vi "MGCC_main_v2.vi"() -> ()   [LabVIEW 2016]
uses:
  <vilib>/imath/engines/lvmath2/RunTimeEngine/IndexRead/NIMS V(S).vi
  <instcachedir>/0/NIMS V(S)_0488751826AF41519A22953C041130DC.lvgen/NIMS V(S)_0488751826AF41519A22953C041130DC_003.vi
  <vilib>/imathl/engines/lvmath/Functions/Error Handling/Create Error.vi
  <vilib>/imath/engines/lvmath2/RunTimeEngine/NodeEndStatement/NIMS_NodeEndStatement_Output.vi
  <instcachedir>/0/NIMS_NodeEndStatement_Output_53EC0D466D134D7ABD903AC30B43404B.lvgen/NIMS_NodeEndStatement_Output_53EC0D466D134D7ABD903AC30B43404B_011.vi
  <vilib>/imath/engines/lvmath2/RunTimeEngine/ErrorHandling/NIMS_Finalize Error.vi
panel:
  in  "Manual turn off":bool
  in  "Event Manual panel":bool
  out "Function":bool[](array[boolean])
  out "Name_Function":string[](array[string])
  out "State":bool[](array[boolean])
  out "Name of state":string[](array[string])
  out "Current State":string
  out "Next State":string
  out "date/time string":string
  out "Boolean 4":bool
  out "Boolean 3":bool
  out "Boolean 2":bool
  out "Boolean":bool
  in  "Combo Box":string(combo)="State1"
  # "Interrupts"
  # "Finte State Machine"
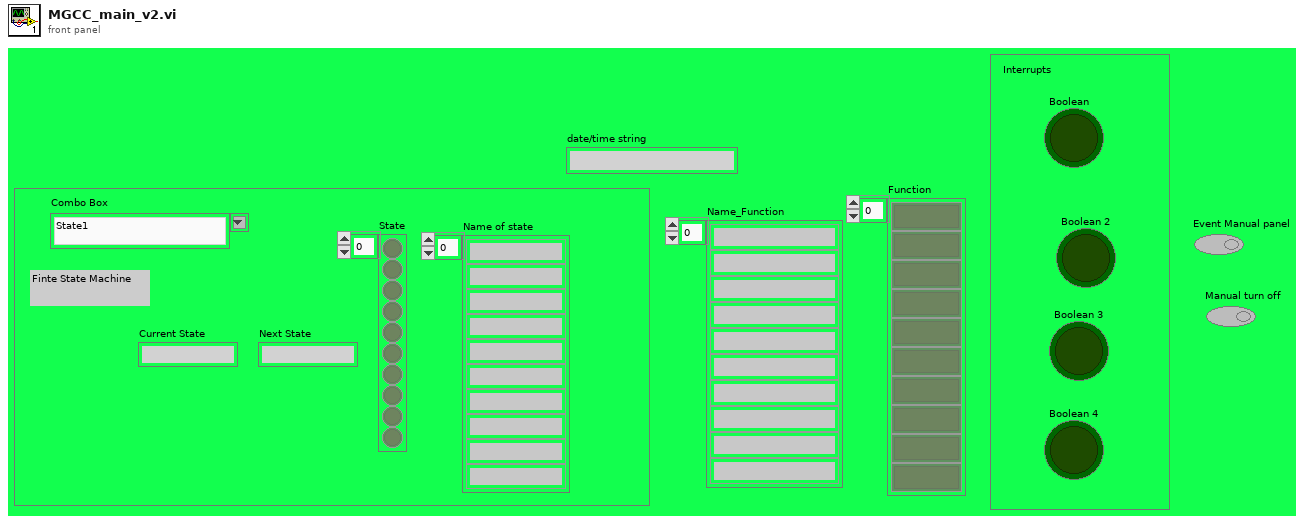
[diagram p1: front panel]
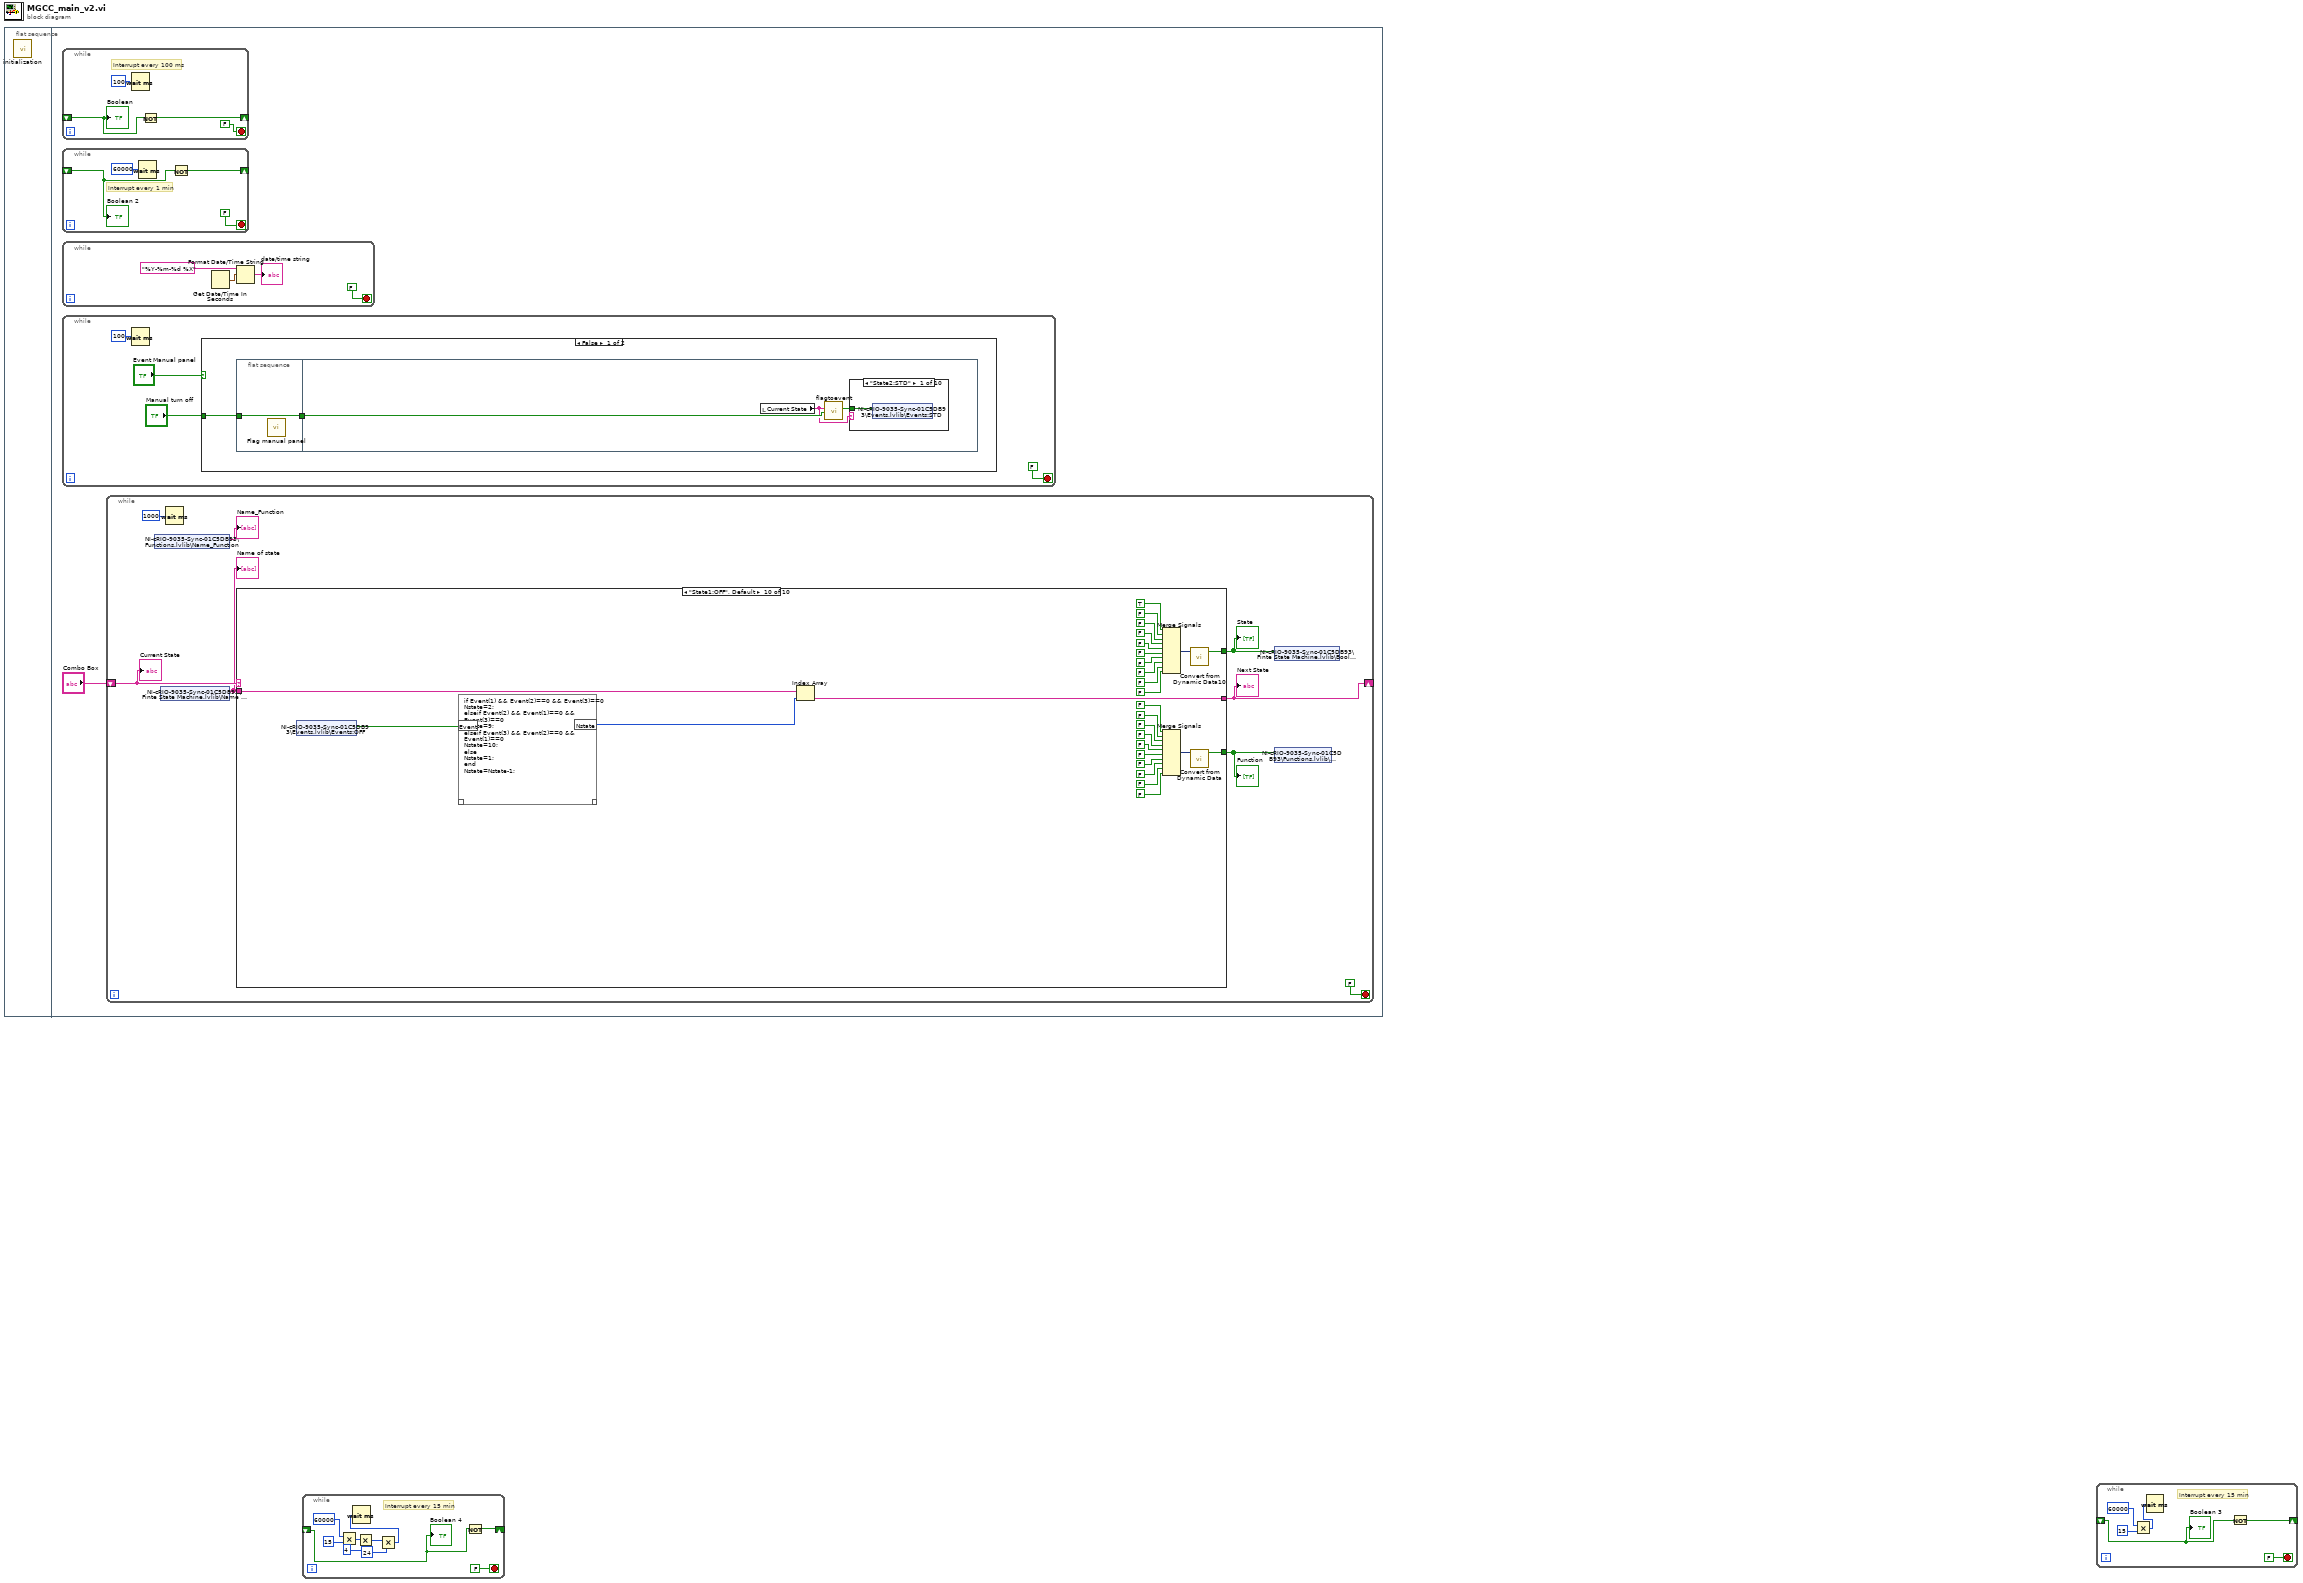
[diagram p0: block diagram]
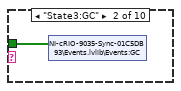
[diagram p2: hidden frame]
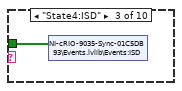
[diagram p3: hidden frame]
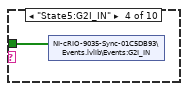
[diagram p4: hidden frame]
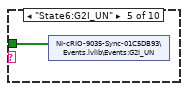
[diagram p5: hidden frame]
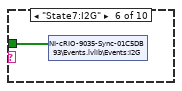
[diagram p6: hidden frame]
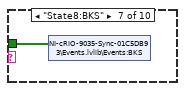
[diagram p7: hidden frame]
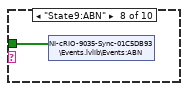
[diagram p8: hidden frame]
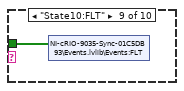
[diagram p9: hidden frame]
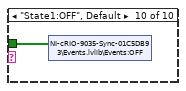
[diagram p10: hidden frame]
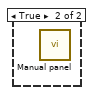
[diagram p11: hidden frame]
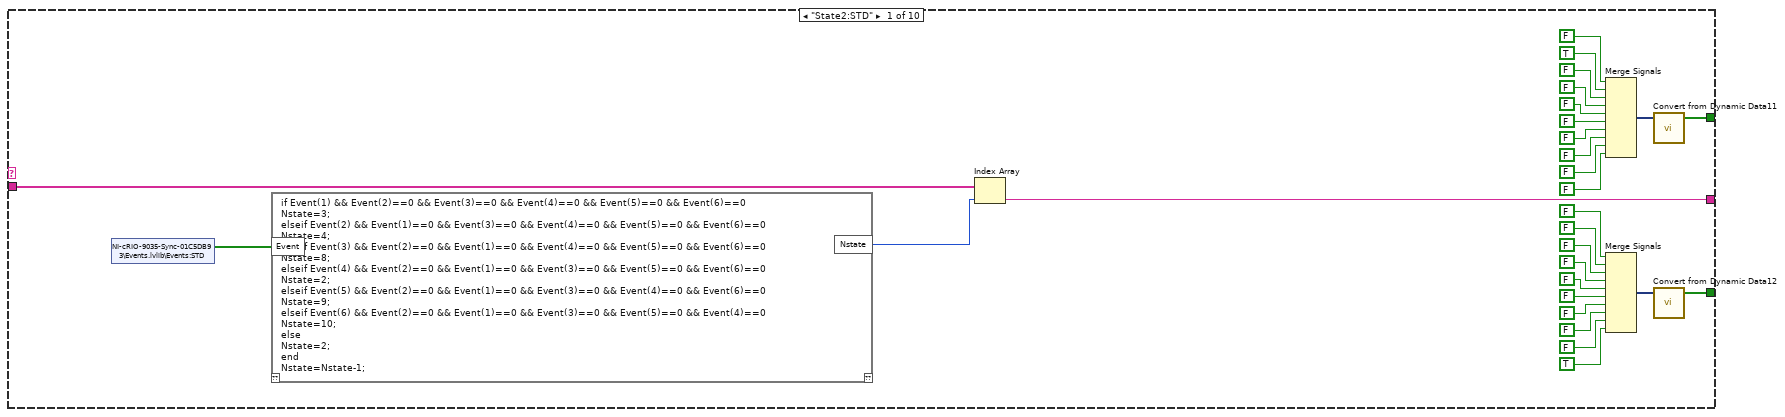
[diagram p12: hidden frame]
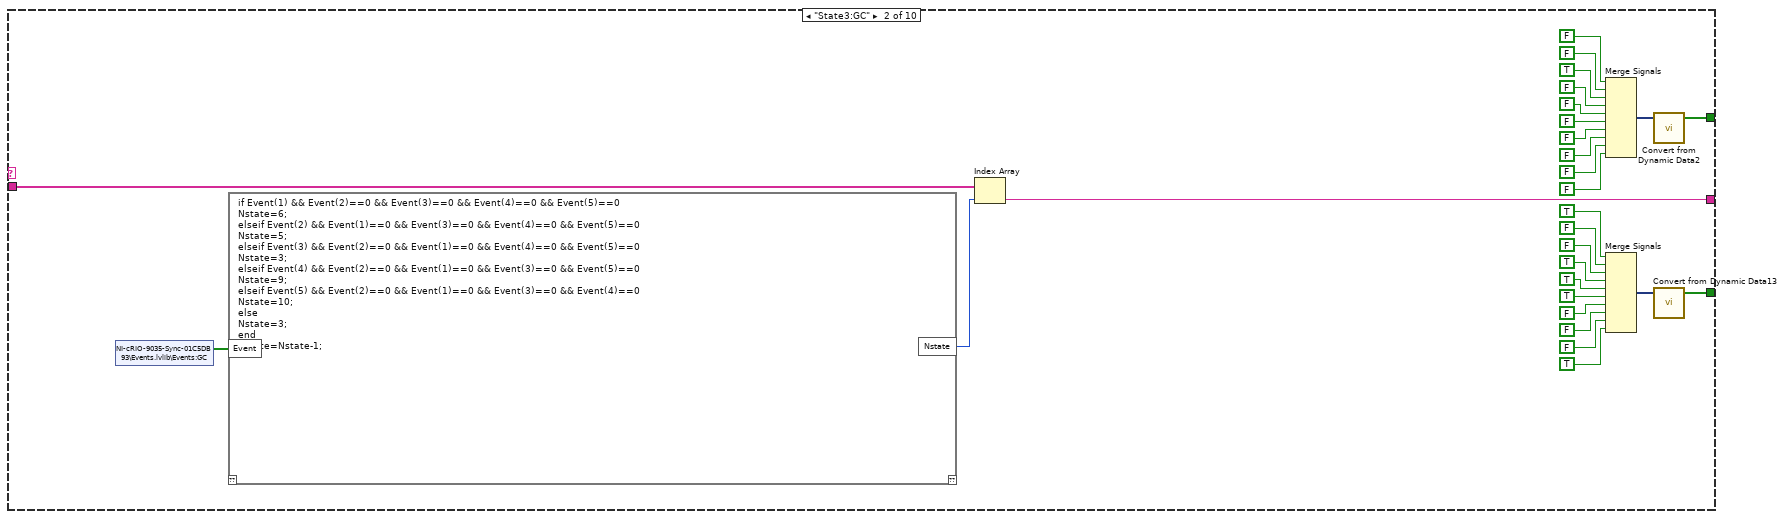
[diagram p13: hidden frame]
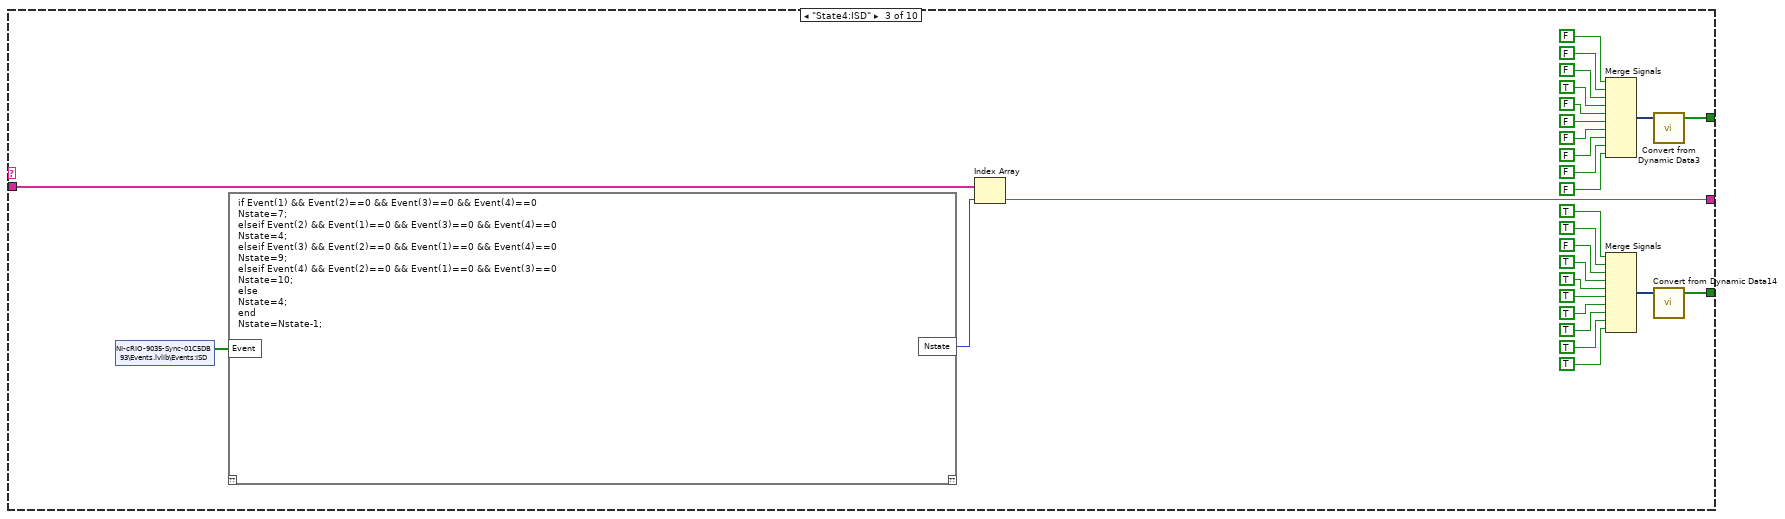
[diagram p14: hidden frame]
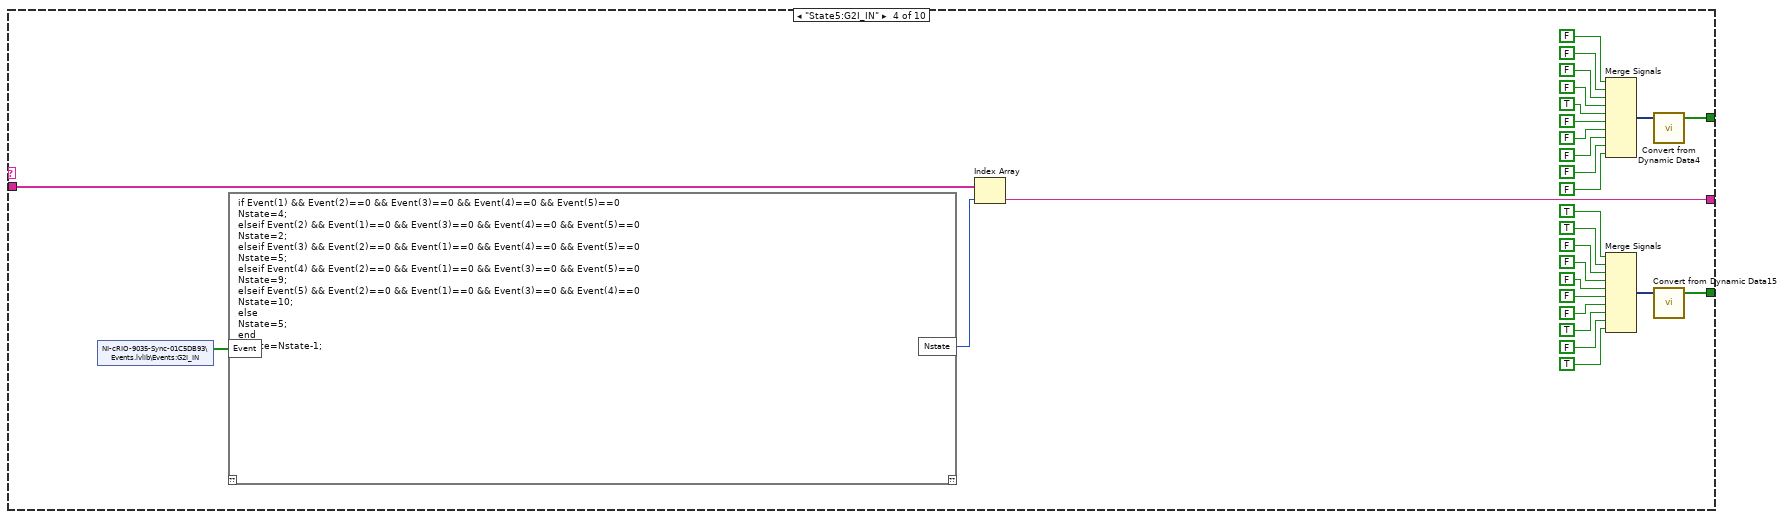
[diagram p15: hidden frame]
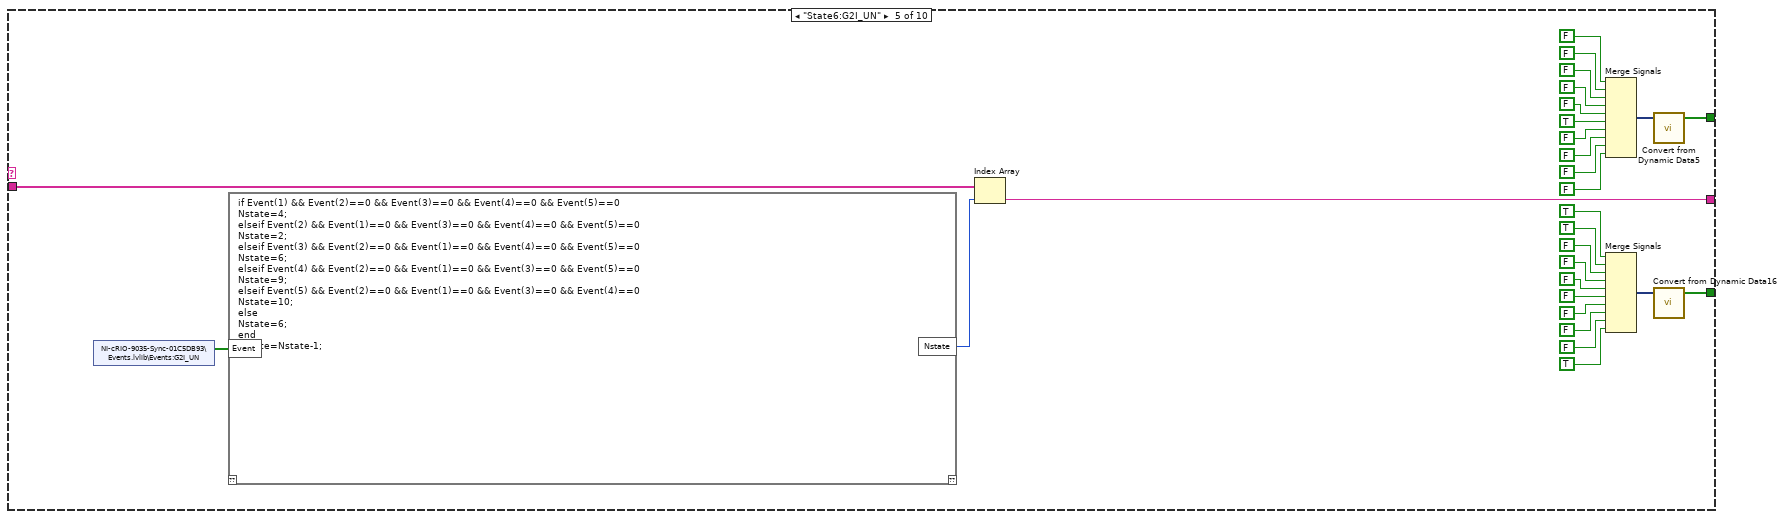
[diagram p16: hidden frame]
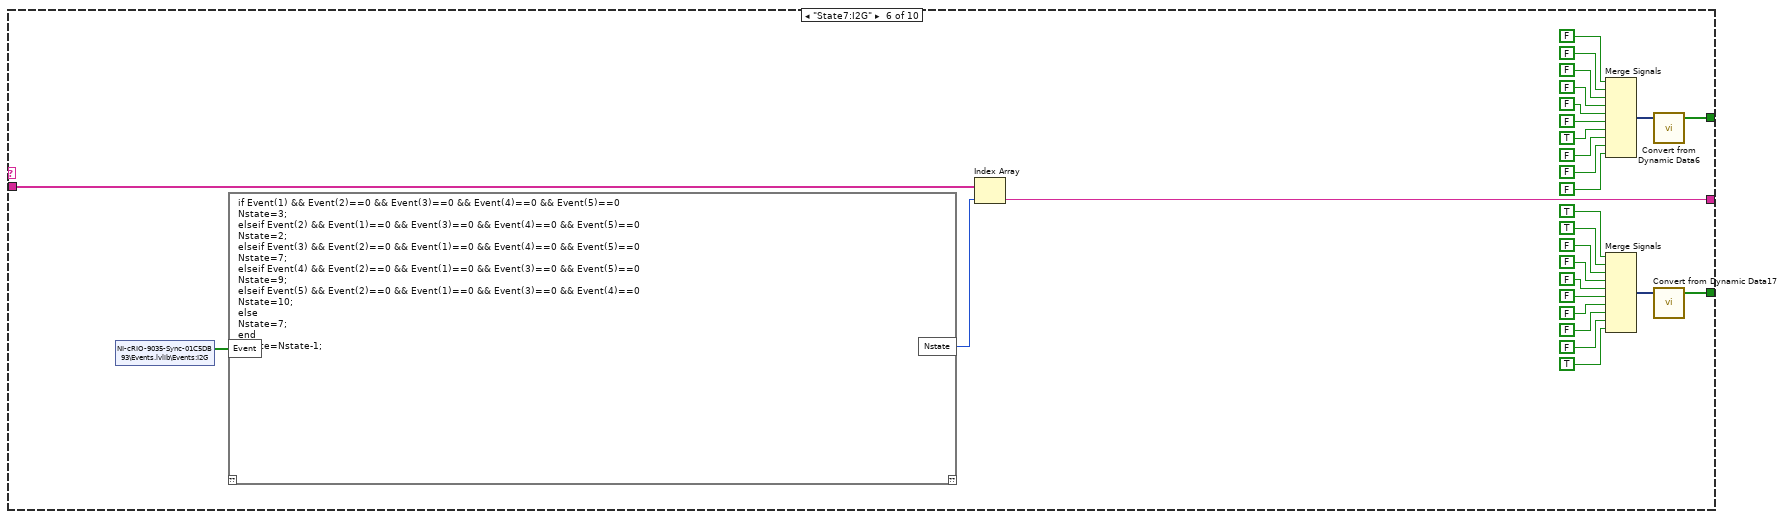
[diagram p17: hidden frame]
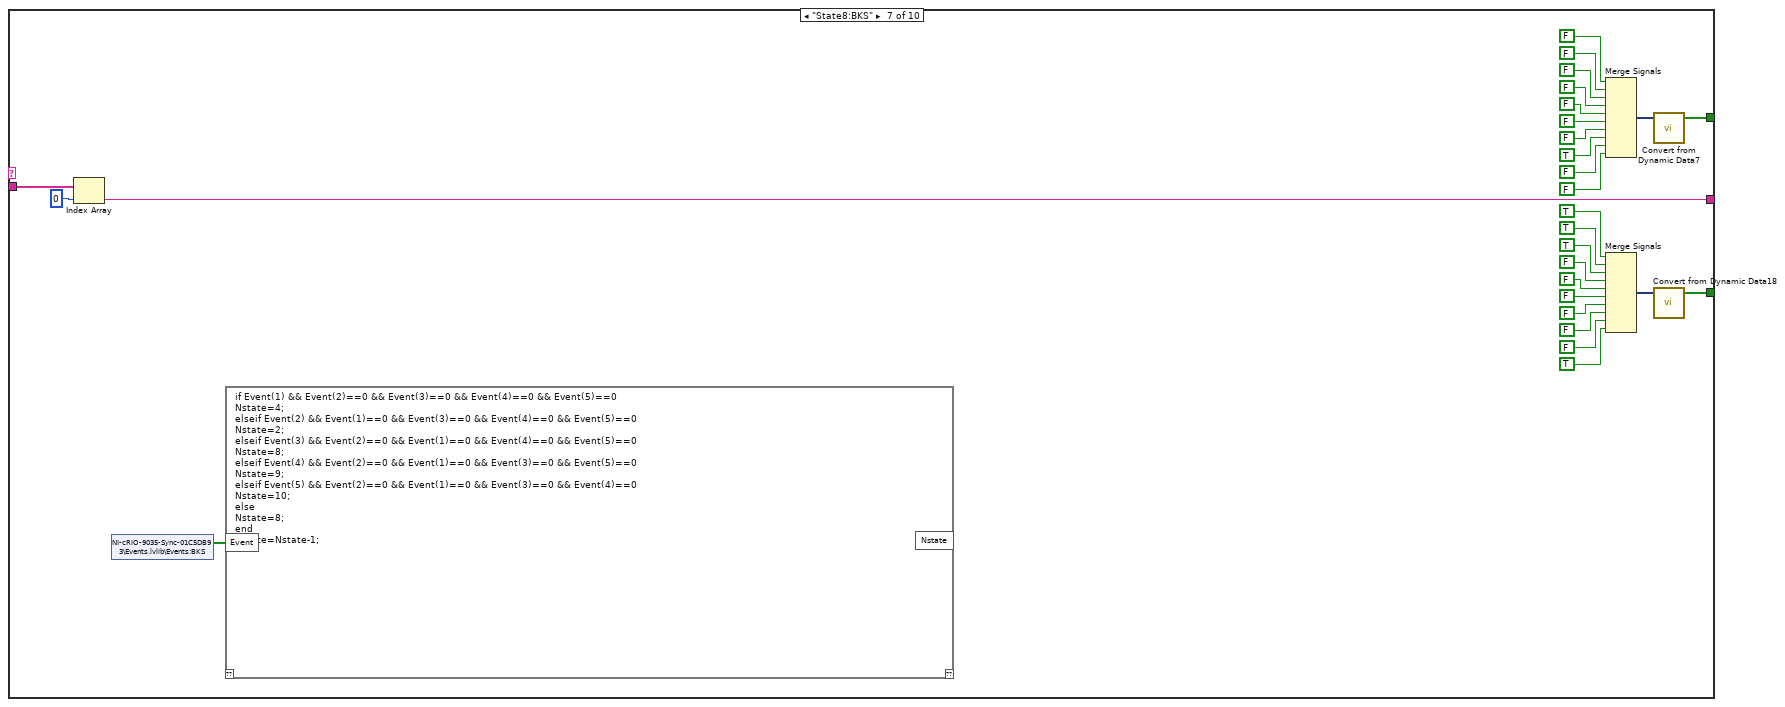
[diagram p18: hidden frame]
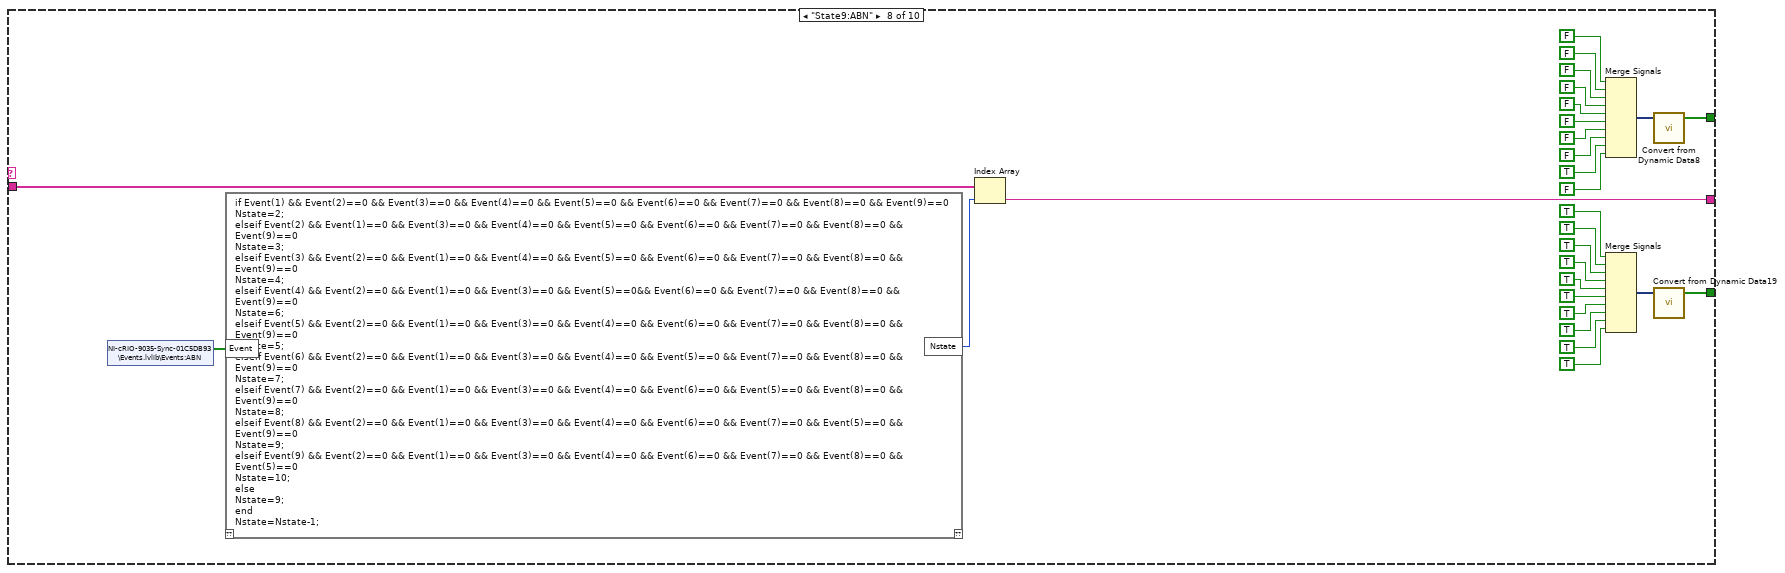
[diagram p19: hidden frame]
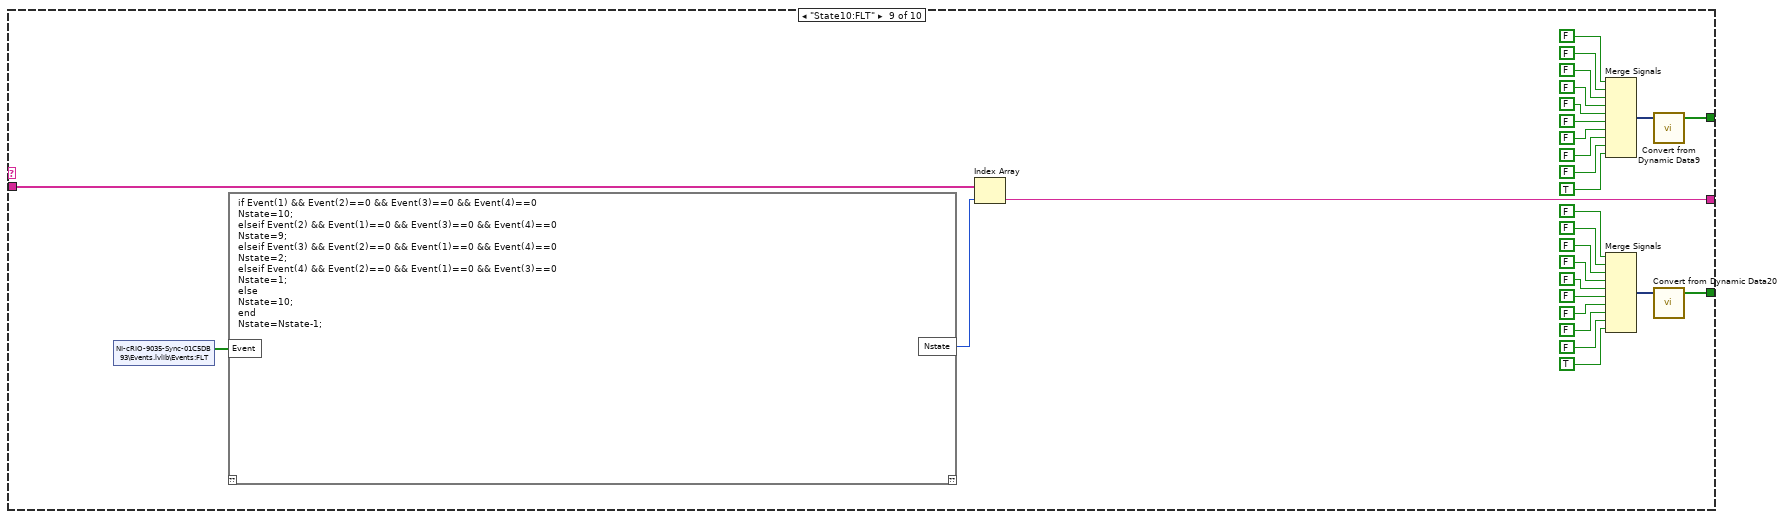
[diagram p20: hidden frame]
diagram:
  n1 = flat-sequence {
    frame #0 {
      n2 = call "initialization.vi"() -> ()  [unwired: 12 in]
    }
    frame #1 {
      n3 = while {
        shift-right: [w31] -> _
        shift-left: _ -> [w32]
        stop <- FALSE stop-if-true
        # "Interrupt every 100 ms"
        n4 = Wait (ms)(milliseconds to wait=u32 100) -> ()  [unwired: 1 out]
        n5 = Not(x=w32) -> (.not. x?=w31:bool)
        "Boolean" <- w32
      }
      n6 = while {
        shift-right: [w28] -> _
        shift-left: _ -> [w27]
        stop <- FALSE stop-if-true
        # "Interrupt every 1 min"
        n7 = Wait (ms)(milliseconds to wait=u32 60000) -> ()  [unwired: 1 out]
        n8 = Not(x=w27) -> (.not. x?=w28:bool)
        "Boolean 2" <- w27
      }
      n9 = while {
        stop <- FALSE stop-if-true
        n10 = Get Date/Time In Seconds() -> (seconds since 1Jan1904=w24:timestamp)
        n11 = Format Date/Time String(time format string (%c)="%Y-%m-%d %X", seconds (now)=w24) -> (date/time string=→"date/time string":string)  [unwired: 1 in]
      }
      n12 = while {
        stop <- FALSE stop-if-true
        n13 = Wait (ms)(milliseconds to wait=u32 100) -> ()  [unwired: 1 out]
        n14 = case shown="False" "Event Manual panel" {
          tunnel: "Manual turn off" -> [w7 _]
          frame False {
            n15 = flat-sequence {
              tunnel: w7 -> [w8]
              tunnel: [w8] -> w6
              tunnel: w6 -> [w11]
              frame #0 {
                n16 = call "Flag manual panel.vi"() -> ()  [unwired: 12 in]
              }
              frame #1 {
                n17 = local read "Current State"() -> (w9:string)
                n18 = call "flagtoevent.vi"("M_OFF"=w11, "Pre_state"=w9) -> ("Event"=w10:bool[])  [unwired: 9 in]
                n19 = case shown="\"State2:STD\"" w9 {
                  tunnel: w10 -> [w12 w13 w14 w15 w16 w17 w18 w19 w20 w21]
                  frame "State2:STD" {
                    n20 = shared-variable "NI-cRIO-9035-Sync-01C5DB93\\Events.lvlib\\Events:STD"(w12) -> ()  [unwired: 1 in, 1 out]
                  }
                  frame "State3:GC" {
                    n21 = shared-variable "NI-cRIO-9035-Sync-01C5DB93\\Events.lvlib\\Events:GC"(w13) -> ()  [unwired: 1 in, 1 out]
                  }
                  frame "State4:ISD" {
                    n22 = shared-variable "NI-cRIO-9035-Sync-01C5DB93\\Events.lvlib\\Events:ISD"(w14) -> ()  [unwired: 1 in, 1 out]
                  }
                  frame "State5:G2I_IN" {
                    n23 = shared-variable "NI-cRIO-9035-Sync-01C5DB93\\Events.lvlib\\Events:G2I_IN"(w15) -> ()  [unwired: 1 in, 1 out]
                  }
                  frame "State6:G2I_UN" {
                    n24 = shared-variable "NI-cRIO-9035-Sync-01C5DB93\\Events.lvlib\\Events:G2I_UN"(w16) -> ()  [unwired: 1 in, 1 out]
                  }
                  frame "State7:I2G" {
                    n25 = shared-variable "NI-cRIO-9035-Sync-01C5DB93\\Events.lvlib\\Events:I2G"(w17) -> ()  [unwired: 1 in, 1 out]
                  }
                  frame "State8:BKS" {
                    n26 = shared-variable "NI-cRIO-9035-Sync-01C5DB93\\Events.lvlib\\Events:BKS"(w18) -> ()  [unwired: 1 in, 1 out]
                  }
                  frame "State9:ABN" {
                    n27 = shared-variable "NI-cRIO-9035-Sync-01C5DB93\\Events.lvlib\\Events:ABN"(w19) -> ()  [unwired: 1 in, 1 out]
                  }
                  frame "State10:FLT" {
                    n28 = shared-variable "NI-cRIO-9035-Sync-01C5DB93\\Events.lvlib\\Events:FLT"(w20) -> ()  [unwired: 1 in, 1 out]
                  }
                  frame "State1:OFF", Default {
                    n29 = shared-variable "NI-cRIO-9035-Sync-01C5DB93\\Events.lvlib\\Events:OFF"(w21) -> ()  [unwired: 1 in, 1 out]
                  }
                }
              }
            }
          }
          frame True {
            n30 = call "Manual panel.vi"() -> ()  [unwired: 12 in]
          }
        }
      }
      n31 = while {
        shift-right: [w40] -> _
        shift-left: "Combo Box" -> [w41]
        stop <- FALSE stop-if-true
        n32 = shared-variable "NI-cRIO-9035-Sync-01C5DB93\\Functions.lvlib\\Name_Function"() -> (→"Name_Function":string[])  [unwired: 1 in, 1 out]
        n33 = shared-variable "NI-cRIO-9035-Sync-01C5DB93\\Finte State Machine.lvlib\\Name of state"() -> (w37:string[])  [unwired: 1 in, 1 out]
        "Name of state" <- w37
        n34 = Wait (ms)(milliseconds to wait=u32 1000) -> ()  [unwired: 1 out]
        n35 = case shown="\"State1:OFF\", Default" w41 {
          tunnel: [w69 w1036 w1735 w2204 w2903 w3602 w4300 w5000 w7119 w7600] -> w40
          tunnel: [w57 w1037 w1736 w2205 w2904 w3603 w4302 w5001 w7120 w7588] -> w36
          tunnel: w37 -> [w56 w1035 w1734 w2203 w2902 w3601 w4299 w4999 w7118 w7587]
          tunnel: [w42 w1021 w1720 w2189 w2888 w3587 w4286 w4985 w7104 w7573] -> w35
          frame "State2:STD" {
            n36 = shared-variable "NI-cRIO-9035-Sync-01C5DB93\\Events.lvlib\\Events:STD"() -> (w55:bool[])  [unwired: 1 in, 1 out]
            n37 = mathscript code="if Event(1) && Event(2)==0 && Event(3)==0 && Event(4)==0 && Event(5)==0 && Event(6)==0\nNstate=3;\nelseif Event(2) && Event(1)==0 && Event(3)==0 && Event(4)==0 && Event(5)==0 && Event(6)==0\nNstate=4;\nelseif Event(3) && Event(2)==0 && Event(1)==0 && Event(4)==0 && Event(5)==0 && Event(6)==0\nNstate=8;\nelseif Event(4) && Event(2)==0 && Event(1)==0 && Event(3)==0 && Event(5)==0 && Event(6)==0\nNstate=2;\nelseif Event(5) && Event(2)==0 && Event(1)==0 && Event(3)==0 && Event(4)==0 && Event(6)==0\nNstate=9;\nelseif Event(6) && Event(2)==0 && Event(1)==0 && Event(3)==0 && Event(5)==0 && Event(4)==0\nNstate=10;\nelse\nNstate=2;\nend\nNstate=Nstate-1;"("Event"=w55) -> ("Nstate"=w54:i32)  [unwired: 1 in, 1 out]
            n38 = Index Array(array=w56, index=w54) -> (element=w69:string)
            n39 = Merge Signals(FALSE ("State3"), TRUE ("State3"), FALSE ("State3"), FALSE ("State3"), FALSE ("State3"), FALSE ("State3"), FALSE ("State3"), FALSE ("State3"), FALSE ("State3"), FALSE ("State3")) -> (w58:dynamicdata)
            n40 = Merge Signals(FALSE ("State3"), FALSE ("State3"), FALSE ("State3"), FALSE ("State3"), FALSE ("State3"), FALSE ("State3"), FALSE ("State3"), FALSE ("State3"), FALSE ("State3"), TRUE ("State3")) -> (w43:dynamicdata)
            n41 = call "Convert from Dynamic Data11"("Dynamic Data Type"=w58) -> ("Array"=w57:bool[])  [unwired: 3 in]
            n42 = call "Convert from Dynamic Data12"("Dynamic Data Type"=w43) -> ("Array"=w42:bool[])  [unwired: 3 in]
          }
          frame "State3:GC" {
            n43 = shared-variable "NI-cRIO-9035-Sync-01C5DB93\\Events.lvlib\\Events:GC"() -> (w1034:bool[])  [unwired: 1 in, 1 out]
            n44 = mathscript code="if Event(1) && Event(2)==0 && Event(3)==0 && Event(4)==0 && Event(5)==0 \nNstate=6;\nelseif Event(2) && Event(1)==0 && Event(3)==0 && Event(4)==0 && Event(5)==0 \nNstate=5;\nelseif Event(3) && Event(2)==0 && Event(1)==0 && Event(4)==0 && Event(5)==0 \nNstate=3;\nelseif Event(4) && Event(2)==0 && Event(1)==0 && Event(3)==0 && Event(5)==0\nNstate=9;\nelseif Event(5) && Event(2)==0 && Event(1)==0 && Event(3)==0 && Event(4)==0 \nNstate=10;\nelse\nNstate=3;\nend\nNstate=Nstate-1;"("Event"=w1034) -> ("Nstate"=w1033:i32)  [unwired: 1 in, 1 out]
            n45 = Index Array(array=w1035, index=w1033) -> (element=w1036:string)
            n46 = Merge Signals(FALSE ("State3"), FALSE ("State3"), TRUE ("State3"), FALSE ("State3"), FALSE ("State3"), FALSE ("State3"), FALSE ("State3"), FALSE ("State3"), FALSE ("State3"), FALSE ("State3")) -> (w1038:dynamicdata)
            n47 = Merge Signals(TRUE ("State3"), FALSE ("State3"), FALSE ("State3"), TRUE ("State3"), TRUE ("State3"), TRUE ("State3"), FALSE ("State3"), FALSE ("State3"), FALSE ("State3"), TRUE ("State3")) -> (w1022:dynamicdata)
            n48 = call "Convert from Dynamic Data2"("Dynamic Data Type"=w1038) -> ("Array"=w1037:bool[])  [unwired: 3 in]
            n49 = call "Convert from Dynamic Data13"("Dynamic Data Type"=w1022) -> ("Array"=w1021:bool[])  [unwired: 3 in]
          }
          frame "State4:ISD" {
            n50 = shared-variable "NI-cRIO-9035-Sync-01C5DB93\\Events.lvlib\\Events:ISD"() -> (w1733:bool[])  [unwired: 1 in, 1 out]
            n51 = mathscript code="if Event(1) && Event(2)==0 && Event(3)==0 && Event(4)==0 \nNstate=7;\nelseif Event(2) && Event(1)==0 && Event(3)==0 && Event(4)==0 \nNstate=4;\nelseif Event(3) && Event(2)==0 && Event(1)==0 && Event(4)==0 \nNstate=9;\nelseif Event(4) && Event(2)==0 && Event(1)==0 && Event(3)==0 \nNstate=10;\nelse\nNstate=4;\nend\nNstate=Nstate-1;"("Event"=w1733) -> ("Nstate"=w1732:i32)  [unwired: 1 in, 1 out]
            n52 = Index Array(array=w1734, index=w1732) -> (element=w1735:string)
            n53 = Merge Signals(FALSE ("State3"), FALSE ("State3"), FALSE ("State3"), TRUE ("State3"), FALSE ("State3"), FALSE ("State3"), FALSE ("State3"), FALSE ("State3"), FALSE ("State3"), FALSE ("State3")) -> (w1737:dynamicdata)
            n54 = Merge Signals(TRUE ("State3"), TRUE ("State3"), FALSE ("State3"), TRUE ("State3"), TRUE ("State3"), TRUE ("State3"), TRUE ("State3"), TRUE ("State3"), TRUE ("State3"), TRUE ("State3")) -> (w1721:dynamicdata)
            n55 = call "Convert from Dynamic Data3"("Dynamic Data Type"=w1737) -> ("Array"=w1736:bool[])  [unwired: 3 in]
            n56 = call "Convert from Dynamic Data14"("Dynamic Data Type"=w1721) -> ("Array"=w1720:bool[])  [unwired: 3 in]
          }
          frame "State5:G2I_IN" {
            n57 = shared-variable "NI-cRIO-9035-Sync-01C5DB93\\Events.lvlib\\Events:G2I_IN"() -> (w2202:bool[])  [unwired: 1 in, 1 out]
            n58 = mathscript code="if Event(1) && Event(2)==0 && Event(3)==0 && Event(4)==0 && Event(5)==0 \nNstate=4;\nelseif Event(2) && Event(1)==0 && Event(3)==0 && Event(4)==0 && Event(5)==0 \nNstate=2;\nelseif Event(3) && Event(2)==0 && Event(1)==0 && Event(4)==0 && Event(5)==0 \nNstate=5;\nelseif Event(4) && Event(2)==0 && Event(1)==0 && Event(3)==0 && Event(5)==0\nNstate=9;\nelseif Event(5) && Event(2)==0 && Event(1)==0 && Event(3)==0 && Event(4)==0 \nNstate=10;\nelse\nNstate=5;\nend\nNstate=Nstate-1;"("Event"=w2202) -> ("Nstate"=w2201:i32)  [unwired: 1 in, 1 out]
            n59 = Index Array(array=w2203, index=w2201) -> (element=w2204:string)
            n60 = Merge Signals(FALSE ("State3"), FALSE ("State3"), FALSE ("State3"), FALSE ("State3"), TRUE ("State3"), FALSE ("State3"), FALSE ("State3"), FALSE ("State3"), FALSE ("State3"), FALSE ("State3")) -> (w2206:dynamicdata)
            n61 = Merge Signals(TRUE ("State3"), TRUE ("State3"), FALSE ("State3"), FALSE ("State3"), FALSE ("State3"), FALSE ("State3"), FALSE ("State3"), TRUE ("State3"), FALSE ("State3"), TRUE ("State3")) -> (w2190:dynamicdata)
            n62 = call "Convert from Dynamic Data4"("Dynamic Data Type"=w2206) -> ("Array"=w2205:bool[])  [unwired: 3 in]
            n63 = call "Convert from Dynamic Data15"("Dynamic Data Type"=w2190) -> ("Array"=w2189:bool[])  [unwired: 3 in]
          }
          frame "State6:G2I_UN" {
            n64 = shared-variable "NI-cRIO-9035-Sync-01C5DB93\\Events.lvlib\\Events:G2I_UN"() -> (w2900:bool[])  [unwired: 1 in, 1 out]
            n65 = mathscript code="if Event(1) && Event(2)==0 && Event(3)==0 && Event(4)==0 && Event(5)==0 \nNstate=4;\nelseif Event(2) && Event(1)==0 && Event(3)==0 && Event(4)==0 && Event(5)==0 \nNstate=2;\nelseif Event(3) && Event(2)==0 && Event(1)==0 && Event(4)==0 && Event(5)==0 \nNstate=6;\nelseif Event(4) && Event(2)==0 && Event(1)==0 && Event(3)==0 && Event(5)==0\nNstate=9;\nelseif Event(5) && Event(2)==0 && Event(1)==0 && Event(3)==0 && Event(4)==0 \nNstate=10;\nelse\nNstate=6;\nend\nNstate=Nstate-1;"("Event"=w2900) -> ("Nstate"=w2901:i32)  [unwired: 1 in, 1 out]
            n66 = Index Array(array=w2902, index=w2901) -> (element=w2903:string)
            n67 = Merge Signals(FALSE ("State3"), FALSE ("State3"), FALSE ("State3"), FALSE ("State3"), FALSE ("State3"), TRUE ("State3"), FALSE ("State3"), FALSE ("State3"), FALSE ("State3"), FALSE ("State3")) -> (w2905:dynamicdata)
            n68 = Merge Signals(TRUE ("State3"), TRUE ("State3"), FALSE ("State3"), FALSE ("State3"), FALSE ("State3"), FALSE ("State3"), FALSE ("State3"), FALSE ("State3"), FALSE ("State3"), TRUE ("State3")) -> (w2889:dynamicdata)
            n69 = call "Convert from Dynamic Data5"("Dynamic Data Type"=w2905) -> ("Array"=w2904:bool[])  [unwired: 3 in]
            n70 = call "Convert from Dynamic Data16"("Dynamic Data Type"=w2889) -> ("Array"=w2888:bool[])  [unwired: 3 in]
          }
          frame "State7:I2G" {
            n71 = shared-variable "NI-cRIO-9035-Sync-01C5DB93\\Events.lvlib\\Events:I2G"() -> (w3599:bool[])  [unwired: 1 in, 1 out]
            n72 = mathscript code="if Event(1) && Event(2)==0 && Event(3)==0 && Event(4)==0 && Event(5)==0 \nNstate=3;\nelseif Event(2) && Event(1)==0 && Event(3)==0 && Event(4)==0 && Event(5)==0 \nNstate=2;\nelseif Event(3) && Event(2)==0 && Event(1)==0 && Event(4)==0 && Event(5)==0 \nNstate=7;\nelseif Event(4) && Event(2)==0 && Event(1)==0 && Event(3)==0 && Event(5)==0\nNstate=9;\nelseif Event(5) && Event(2)==0 && Event(1)==0 && Event(3)==0 && Event(4)==0 \nNstate=10;\nelse\nNstate=7;\nend\nNstate=Nstate-1;"("Event"=w3599) -> ("Nstate"=w3600:i32)  [unwired: 1 in, 1 out]
            n73 = Index Array(array=w3601, index=w3600) -> (element=w3602:string)
            n74 = Merge Signals(FALSE ("State3"), FALSE ("State3"), FALSE ("State3"), FALSE ("State3"), FALSE ("State3"), FALSE ("State3"), TRUE ("State3"), FALSE ("State3"), FALSE ("State3"), FALSE ("State3")) -> (w3604:dynamicdata)
            n75 = Merge Signals(TRUE ("State3"), TRUE ("State3"), FALSE ("State3"), FALSE ("State3"), FALSE ("State3"), FALSE ("State3"), FALSE ("State3"), FALSE ("State3"), FALSE ("State3"), TRUE ("State3")) -> (w3588:dynamicdata)
            n76 = call "Convert from Dynamic Data6"("Dynamic Data Type"=w3604) -> ("Array"=w3603:bool[])  [unwired: 3 in]
            n77 = call "Convert from Dynamic Data17"("Dynamic Data Type"=w3588) -> ("Array"=w3587:bool[])  [unwired: 3 in]
          }
          frame "State8:BKS" {
            n78 = Index Array(array=w4299, index=0) -> (element=w4300:string)
            n79 = shared-variable "NI-cRIO-9035-Sync-01C5DB93\\Events.lvlib\\Events:BKS"() -> (w4298:bool[])  [unwired: 1 in, 1 out]
            n80 = mathscript code="if Event(1) && Event(2)==0 && Event(3)==0 && Event(4)==0 && Event(5)==0 \nNstate=4;\nelseif Event(2) && Event(1)==0 && Event(3)==0 && Event(4)==0 && Event(5)==0 \nNstate=2;\nelseif Event(3) && Event(2)==0 && Event(1)==0 && Event(4)==0 && Event(5)==0 \nNstate=8;\nelseif Event(4) && Event(2)==0 && Event(1)==0 && Event(3)==0 && Event(5)==0\nNstate=9;\nelseif Event(5) && Event(2)==0 && Event(1)==0 && Event(3)==0 && Event(4)==0 \nNstate=10;\nelse\nNstate=8;\nend\nNstate=Nstate-1;"("Event"=w4298) -> ()  [unwired: 1 in, 2 out]
            n81 = Merge Signals(FALSE ("State3"), FALSE ("State3"), FALSE ("State3"), FALSE ("State3"), FALSE ("State3"), FALSE ("State3"), FALSE ("State3"), TRUE ("State3"), FALSE ("State3"), FALSE ("State3")) -> (w4303:dynamicdata)
            n82 = Merge Signals(TRUE ("State3"), TRUE ("State3"), TRUE ("State3"), FALSE ("State3"), FALSE ("State3"), FALSE ("State3"), FALSE ("State3"), FALSE ("State3"), FALSE ("State3"), TRUE ("State3")) -> (w4287:dynamicdata)
            n83 = call "Convert from Dynamic Data7"("Dynamic Data Type"=w4303) -> ("Array"=w4302:bool[])  [unwired: 3 in]
            n84 = call "Convert from Dynamic Data18"("Dynamic Data Type"=w4287) -> ("Array"=w4286:bool[])  [unwired: 3 in]
          }
          frame "State9:ABN" {
            n85 = shared-variable "NI-cRIO-9035-Sync-01C5DB93\\Events.lvlib\\Events:ABN"() -> (w4998:bool[])  [unwired: 1 in, 1 out]
            n86 = mathscript code="if Event(1) && Event(2)==0 && Event(3)==0 && Event(4)==0 && Event(5)==0 && Event(6)==0 && Event(7)==0 && Event(8)==0 && Event(9)==0 \nNstate=2;\nelseif Event(2) && Event(1)==0 && Event(3)==0 && Event(4)==0 && Event(5)==0 && Event(6)==0 && Event(7)==0 && Event(8)==0 && Event(9)==0 \nNstate=3;\nelseif Event(3) && Event(2)==0 && Event(1)==0 && Event(4)==0 && Event(5)==0 && Event(6)==0 && Event(7)==0 && Event(8)==0 && Event(9)==0 \nNstate=4;\nelseif Event(4) && Event(2)==0 && Event(1)==0 && Event(3)==0 && Event(5)==0&& Event(6)==0 && Event(7)==0 && Event(8)==0 && Event(9)==0 \nNstate=6;\nelseif Event(5) && Event(2)==0 && Event(1)==0 && Event(3)==0 && Event(4)==0 && Event(6)==0 && Event(7)==0 && Event(8)==0 && Event(9)==0 \nNstate=5;\nelseif Event(6) && Event(2)==0 && Event(1)==0 && Event(3)==0 && Event(4)==0 && Event(5)==0 && Event(7)==0 && Event(8)==0 && Event(9)==0 \nNstate=7;\nelseif Event(7) && Event(2)==0 && Event(1)==0 && Event(3)==0 && Event(4)==0 && Event(6)==0 && Event(5)==0 && Event(8)==0 && Event(9)==0 \nNstate=8;\nelseif Event(8) && Event(2)==0 && Event(1)==0 && Event(3)==0 && Event(4)==0 && Event(6)==0 && Event(7)==0 && Event(5)==0 && Event(9)==0 \nNstate=9;\nelseif Event(9) && Event(2)==0 && Event(1)==0 && Event(3)==0 && Event(4)==0 && Event(6)==0 && Event(7)==0 && Event(8)==0 && Event(5)==0 \nNstate=10;\nelse\nNstate=9;\nend\nNstate=Nstate-1;"("Event"=w4998) -> ("Nstate"=w4997:i32)  [unwired: 1 in, 1 out]
            n87 = Index Array(array=w4999, index=w4997) -> (element=w5000:string)
            n88 = Merge Signals(FALSE ("State3"), FALSE ("State3"), FALSE ("State3"), FALSE ("State3"), FALSE ("State3"), FALSE ("State3"), FALSE ("State3"), FALSE ("State3"), TRUE ("State3"), FALSE ("State3")) -> (w5002:dynamicdata)
            n89 = Merge Signals(TRUE ("State3"), TRUE ("State3"), TRUE ("State3"), TRUE ("State3"), TRUE ("State3"), TRUE ("State3"), TRUE ("State3"), TRUE ("State3"), TRUE ("State3"), TRUE ("State3")) -> (w4986:dynamicdata)
            n90 = call "Convert from Dynamic Data8"("Dynamic Data Type"=w5002) -> ("Array"=w5001:bool[])  [unwired: 3 in]
            n91 = call "Convert from Dynamic Data19"("Dynamic Data Type"=w4986) -> ("Array"=w4985:bool[])  [unwired: 3 in]
          }
          frame "State10:FLT" {
            n92 = shared-variable "NI-cRIO-9035-Sync-01C5DB93\\Events.lvlib\\Events:FLT"() -> (w7117:bool[])  [unwired: 1 in, 1 out]
            n93 = mathscript code="if Event(1) && Event(2)==0 && Event(3)==0 && Event(4)==0 \nNstate=10;\nelseif Event(2) && Event(1)==0 && Event(3)==0 && Event(4)==0 \nNstate=9;\nelseif Event(3) && Event(2)==0 && Event(1)==0 && Event(4)==0 \nNstate=2;\nelseif Event(4) && Event(2)==0 && Event(1)==0 && Event(3)==0 \nNstate=1;\nelse\nNstate=10;\nend\nNstate=Nstate-1;"("Event"=w7117) -> ("Nstate"=w7116:i32)  [unwired: 1 in, 1 out]
            n94 = Index Array(array=w7118, index=w7116) -> (element=w7119:string)
            n95 = Merge Signals(FALSE ("State3"), FALSE ("State3"), FALSE ("State3"), FALSE ("State3"), FALSE ("State3"), FALSE ("State3"), FALSE ("State3"), FALSE ("State3"), FALSE ("State3"), TRUE ("State3")) -> (w7121:dynamicdata)
            n96 = Merge Signals(FALSE ("State3"), FALSE ("State3"), FALSE ("State3"), FALSE ("State3"), FALSE ("State3"), FALSE ("State3"), FALSE ("State3"), FALSE ("State3"), FALSE ("State3"), TRUE ("State3")) -> (w7105:dynamicdata)
            n97 = call "Convert from Dynamic Data9"("Dynamic Data Type"=w7121) -> ("Array"=w7120:bool[])  [unwired: 3 in]
            n98 = call "Convert from Dynamic Data20"("Dynamic Data Type"=w7105) -> ("Array"=w7104:bool[])  [unwired: 3 in]
          }
          frame "State1:OFF", Default {
            n99 = shared-variable "NI-cRIO-9035-Sync-01C5DB93\\Events.lvlib\\Events:OFF"() -> (w7586:bool[])  [unwired: 1 in, 1 out]
            n100 = mathscript code="if Event(1) && Event(2)==0 && Event(3)==0\nNstate=2;\nelseif Event(2) && Event(1)==0 && Event(3)==0\nNstate=9;\nelseif Event(3) && Event(2)==0 && Event(1)==0\nNstate=10;\nelse\nNstate=1;\nend\nNstate=Nstate-1;"("Event"=w7586) -> ("Nstate"=w7585:i32)  [unwired: 1 in, 1 out]
            n101 = Index Array(array=w7587, index=w7585) -> (element=w7600:string)
            n102 = Merge Signals(TRUE ("State3"), FALSE ("State3"), FALSE ("State3"), FALSE ("State3"), FALSE ("State3"), FALSE ("State3"), FALSE ("State3"), FALSE ("State3"), FALSE ("State3"), FALSE ("State3")) -> (w7589:dynamicdata)
            n103 = Merge Signals(FALSE ("State3"), FALSE ("State3"), FALSE ("State3"), FALSE ("State3"), FALSE ("State3"), FALSE ("State3"), FALSE ("State3"), FALSE ("State3"), FALSE ("State3"), FALSE ("State3")) -> (w7574:dynamicdata)
            n104 = call "Convert from Dynamic Data10"("Dynamic Data Type"=w7589) -> ("Array"=w7588:bool[])  [unwired: 3 in]
            n105 = call "Convert from Dynamic Data"("Dynamic Data Type"=w7574) -> ("Array"=w7573:bool[])  [unwired: 3 in]
          }
        }
        "Next State" <- w40
        "State" <- w36
        "Function" <- w35
        n106 = shared-variable "NI-cRIO-9035-Sync-01C5DB93\\Finte State Machine.lvlib\\Bool of state"(w36) -> ()  [unwired: 1 in, 1 out]
        n107 = shared-variable "NI-cRIO-9035-Sync-01C5DB93\\Functions.lvlib\\Functions"(w35) -> ()  [unwired: 1 in, 1 out]
        "Current State" <- w41
      }
    }
  }
  n108 = while {
    shift-right: [w7864] -> _
    shift-left: _ -> [w7863]
    stop <- FALSE stop-if-true
    # "Interrupt every 15 min"
    n109 = Multiply(x=u32 60000 ("milliseconds to wait"), y=u32 15) -> (x*y=w7869:u32)
    n110 = Multiply(x=w7869, y=u32 4) -> (x*y=w7868:u32)
    n111 = Multiply(x=w7868, y=u32 24) -> (x*y=w7865:u32)
    n112 = Wait (ms)(milliseconds to wait=w7865) -> ()  [unwired: 1 out]
    n113 = Not(x=w7863) -> (.not. x?=w7864:bool)
    "Boolean 4" <- w7863
  }
  n114 = while {
    shift-right: [w7874] -> _
    shift-left: _ -> [w7873]
    stop <- FALSE stop-if-true
    # "Interrupt every 15 min"
    n115 = Multiply(x=u32 60000 ("milliseconds to wait"), y=u32 15) -> (x*y=w7875:u32)
    n116 = Wait (ms)(milliseconds to wait=w7875) -> ()  [unwired: 1 out]
    n117 = Not(x=w7873) -> (.not. x?=w7874:bool)
    "Boolean 3" <- w7873
  }
